vi "CS_cRIO-PB_DP-Slave_SlaveIOData.vi"(0 "FPGA VI Reference":T1, 7 "Modify input data":u8[](array[numeric]) format="%.0x", 11 "Error":errorcluster) -> (4 "FPGA VI Reference out":T1, 8 "Output data":u8[](array[numeric]) format="%.0x", 10 "Slave status":u8 format="%.0x", 15 "Error out":errorcluster)   [LabVIEW 2013, in "dynamic profibus.lvlib"]
doc: "Handles the cyclic process data of the selected DP-Slave.\n\nFPGA VI Reference:\nReference of the FPGA VI.\n\nSlave:\nPROFIBUS address of the DP-Slave. \n\nModify output data:\nThe Modify output data array contains the DP-Slave output data to be changed.\n\nInput data:\nThe Input data array contains the DP-Slave input data.\n\nOutput data:\nThe Output data array contains the DP-Slave output data.\n\nInput length:\nReturns the configured input length of the DP-Slave.\n\nOutput length:\nReturns the configured output length of the DP-Slave.\n\nSlave status:\n0x00: DP-Slave is in DataExchange mode, input and output data are valid\n0xC3: DP-Slave is not in Data Exchange mode, input and output data are invalid, DP-Slave diagnostic data are reported in Diag data array\n0xFF: DP-Slave is in Data Exchange mode and reports ext. diagnostic data, input and output data are valid.\n\nFPGA VI Reference out:\nIs a copy of the FPGA VI Reference .\n\nError in:\nPreceding error conditions. If an error has already occurred, the VI returns the value of the error in Error out.\n\nError out:\nError: TRUE if an error occurred.\nStatus: Error code\nInfo: Error description"
uses:
  dynamic profibus.lvlib
  CS_cRIO-PB_DP-Slave_FPGA-Reference.ctl
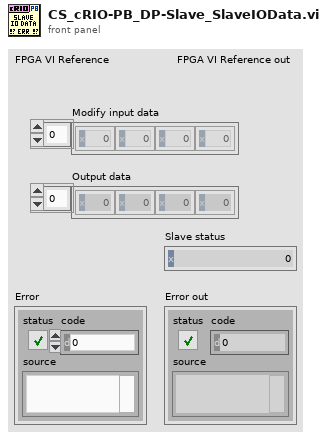
[diagram p1: front panel]
types:
  T1 = typedef "dynamic profibus.lvlib/CS_cRIO-PB_DP-Slave_FPGA-Reference.ctl" = refnum<k20>
  T2 = enum16{"Get DP-AutoSlave Address", "Set DP-AutoSlave Address", "Get Slave Output Data", "Set Slave Input Data", "Read/Write Slave Data"}
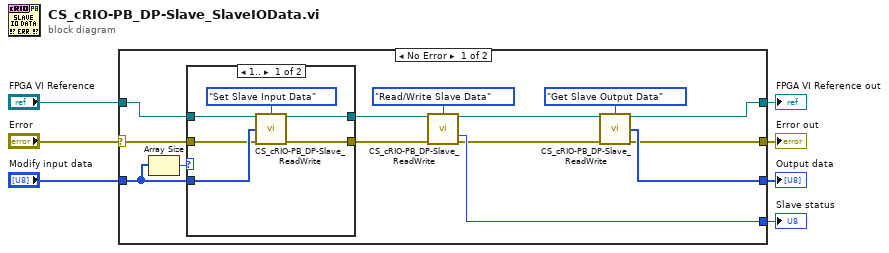
[diagram p0: block diagram]
diagram:
  n1 = case shown="No Error" "Error" {
    selector: "Error" -> [w19 w30]
    tunnel: "FPGA VI Reference" -> [w20 w31]
    tunnel: "Modify input data" -> [w16 _]
    tunnel: [w14 _] -> w4
    tunnel: [w10 w31] -> w3
    tunnel: [w13 w30] -> w2
    tunnel: [w21 _] -> w1
    frame No Error {
      n2 = Array Size(array=w16) -> (size(s)=w15:i32)
      n3 = case shown="1.." w15 {
        tunnel: w16 -> [w25 _]
        tunnel: w20 -> [w24 w28]
        tunnel: w19 -> [w23 w29]
        tunnel: [w27 w29] -> w18
        tunnel: [w26 w28] -> w17
        frame 1.. {
          n4 = call "CS_cRIO-PB_DP-Slave_ReadWrite.vi"("FPGA VI Reference"=w24, "Mode"=T2."Set Slave Input Data", "Data"=w25, "Error"=w23) -> ("FPGA VI Reference out"=w26:T1, "Error out"=w27:errorcluster)  [unwired: 8 in, 2 out]
        }
        frame ..0 {
        }
      }
      n5 = call "CS_cRIO-PB_DP-Slave_ReadWrite.vi"("FPGA VI Reference"=w17, "Mode"=T2."Read/Write Slave Data", "Error"=w18) -> ("FPGA VI Reference out"=w11:T1, "Status"=w21:u8, "Error out"=w12:errorcluster)  [unwired: 9 in, 1 out]
      n6 = call "CS_cRIO-PB_DP-Slave_ReadWrite.vi"("FPGA VI Reference"=w11, "Mode"=T2."Get Slave Output Data", "Error"=w12) -> ("FPGA VI Reference out"=w10:T1, "Data out"=w14:u8[], "Error out"=w13:errorcluster)  [unwired: 9 in, 1 out]
    }
    frame Error {
    }
  }
  "FPGA VI Reference out" <- w3
  "Output data" <- w4
  "Error out" <- w2
  "Slave status" <- w1
